vi "Get Line Name.vi"(8 "error in":errorcluster, 11 "Line in":T1) -> (0 "error out":errorcluster, 2 "Name":string, 3 "Line out":T1)   [LabVIEW 2013, in "tag bus configurable plugin module configuration.lvclass"]
doc: "This VI retrieves the line name or ID, that identifies this element in the cluster, from the line"
uses:
  tag bus configurable plugin module configuration.lvclass
  Line.ctl
  <vilib>/NI/Tag Bus Module Framework/channel/TBM channel.lvclass
  <vilib>/NI/Tag Bus/tag/tag descriptor.lvclass/tag descriptor.ctl
  <vilib>/NI/Tag Bus/tag/tag descriptor.lvclass
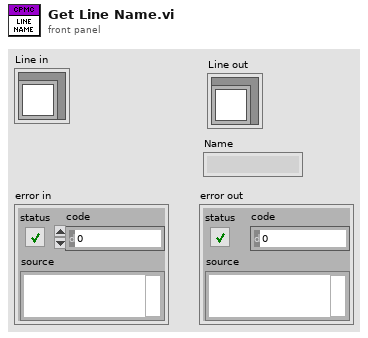
[diagram p1: front panel]
types:
  T1 = typedef "tag bus configurable plugin module configuration.lvclass/Line.ctl" = cluster{"channel":refnum<class "TBM channel.lvclass">}
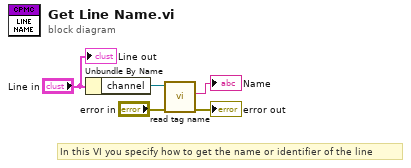
[diagram p0: block diagram]
diagram:
  # "In this VI you specify how to get the name or identifier of the line"
  n1 = Unbundle By Name("Line in") -> ("channel"=w3:refnum<class "TBM channel.lvclass">)
  n2 = call <vilib>:"read tag name.vi"("error in"="error in", "system tag in"=w3) -> ("error out"=→"error out":errorcluster, "name"=→"Name":string)  [unwired: 7 in, 1 out]
  "Line out" <- "Line in"
